vi "ManipEnd.vi"(2 "Time Since Latch":u32, 3 "Instruction String":string) -> (0 "Error Out":errorcluster, 1 "Advance Trigger":bool)   [LabVIEW 2019]
doc: "Stops the subsystem sequencer.\n\nParameters: None"
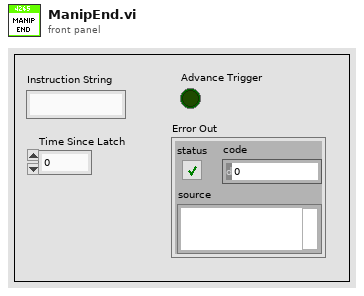
[diagram p1: front panel]
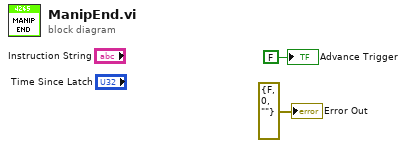
[diagram p0: block diagram]
diagram:
  "Advance Trigger" <- FALSE ("Advance Trigger")
  "Error Out" <- errorcluster {"status"=FALSE, "code"=0, "source"=""} ("error constant")
